vi "Clean Up.vi"(8 "error in (no error)":errorcluster, 11 "MF3 in":refnum<class "MF3.lvclass">) -> (0 "error out":errorcluster, 3 "MF3 out":refnum<class "MF3.lvclass">)   [LabVIEW 2011, in "MF3.lvclass"]
uses:
  MF3.lvclass
  MF3.lvclass/MF3.ctl
  <vilib>/Utility/error.llb/Error Cluster From Error Code.vi
  <vilib>/rvi/errors/niLvFpgaAdjustHostInterfaceError.vi
  <vilib>/FPGAPlugInAG/NI 9157/niLvFpga_Close_NI 9157.vi
  <vilib>/rvi/interface/nirviReadWriteControl/nirviReadWriteControl.xnode
  FPGA/MotorsInterface.lvbitx
  <vilib>/rvi/interface/nirviCloseFPGA/nirviCloseFPGA.xnode
  NiFpgaLv.dll
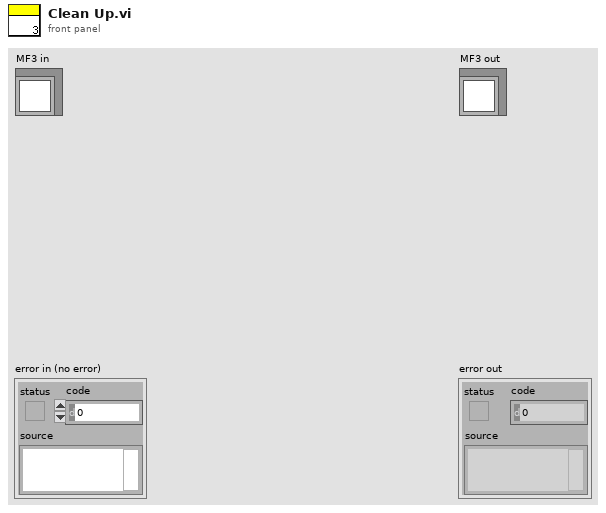
[diagram p1: front panel]
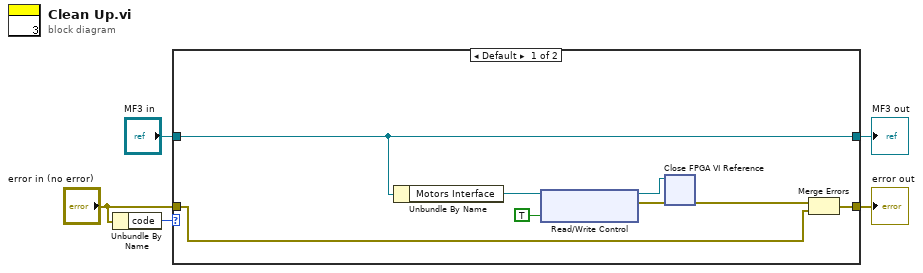
[diagram p0: block diagram]
diagram:
  n1 = Unbundle By Name("error in (no error)") -> ("code"=w3:i32)
  n2 = case shown="Default" w3 {
    tunnel: [w7 w14] -> w1
    tunnel: [w13 w15] -> w4
    tunnel: "MF3 in" -> [w13 w15]
    tunnel: "error in (no error)" -> [w6 w14]
    frame Default {
      n3 = Unbundle By Name(w13) -> ("Motors Interface"=w12:refnum<k20>)
      n4 = xnode "Read/Write Control"("FPGA VI Reference In"=w12, "Disable Motors"=TRUE) -> ("FPGA VI Reference Out"=w10:refnum<k20>, "error out"=w9:errorcluster)  [unwired: 1 in]
      n5 = xnode "Close FPGA VI Reference"("FPGA VI Reference In"=w10, "error in"=w9) -> ("error out"=w8:errorcluster)
      n6 = Merge Errors(w8, w6) -> (w7:errorcluster)
    }
    frame -65536 {
      # "Unable to communicate with the module. Reinsert the module and check connections.\nIf the chassis is in FPGA Interface programming mode, make sure you have opened an \nFPGA reference to a bitfile or FPGA VI with Scan Interface support for the module you are \ntrying to access using the Scan Interface."
    }
  }
  "error out" <- w1
  "MF3 out" <- w4
